vi "2D_Iteration_Data.vi"(9 "Iteration":i32, 10 "ID":dbl) -> (1 "y0":dbl, 2 "x0":dbl)   [LabVIEW 2011]
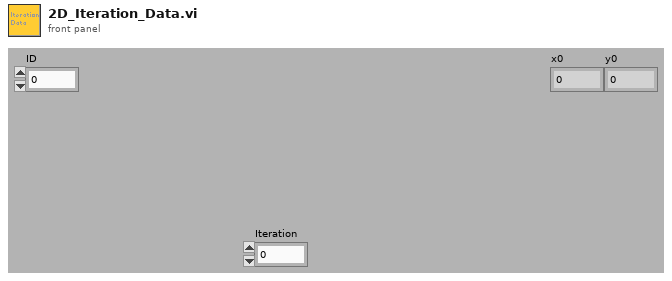
[diagram p1: front panel]
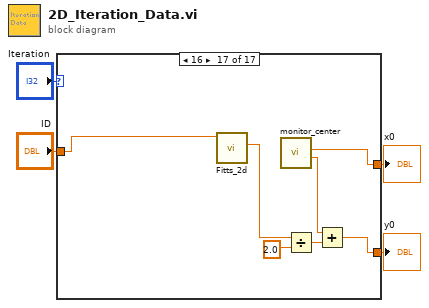
[diagram p0: block diagram]
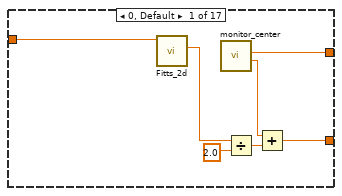
[diagram p2: hidden frame]
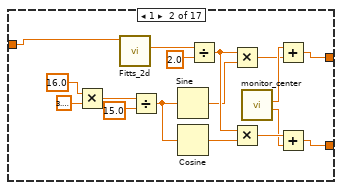
[diagram p3: hidden frame]
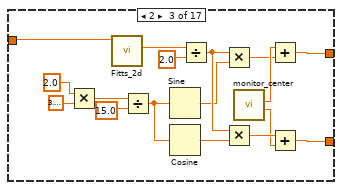
[diagram p4: hidden frame]
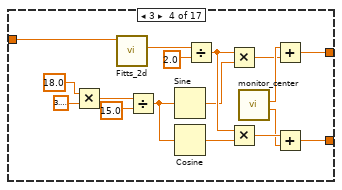
[diagram p5: hidden frame]
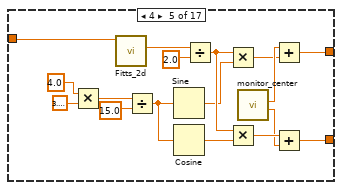
[diagram p6: hidden frame]
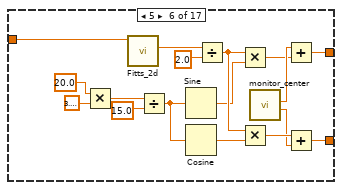
[diagram p7: hidden frame]
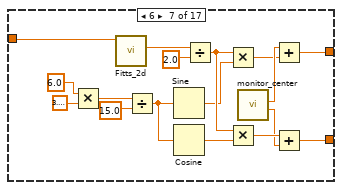
[diagram p8: hidden frame]
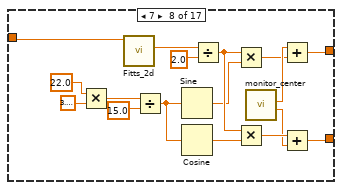
[diagram p9: hidden frame]
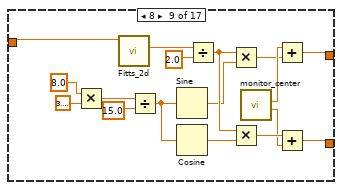
[diagram p10: hidden frame]
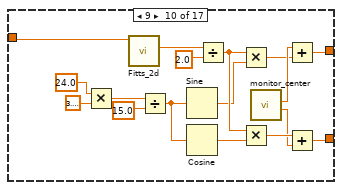
[diagram p11: hidden frame]
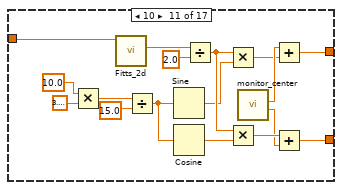
[diagram p12: hidden frame]
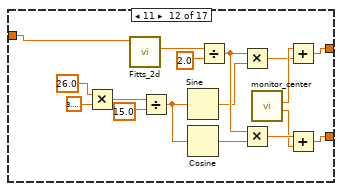
[diagram p13: hidden frame]
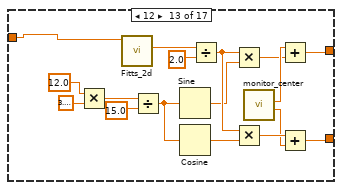
[diagram p14: hidden frame]
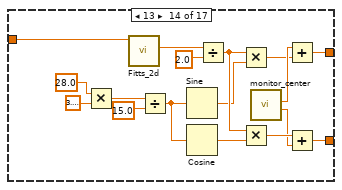
[diagram p15: hidden frame]
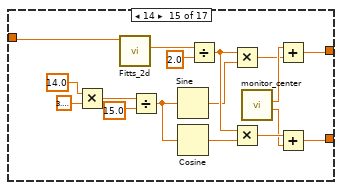
[diagram p16: hidden frame]
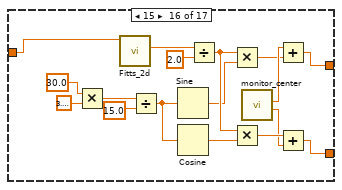
[diagram p17: hidden frame]
diagram:
  n1 = case shown="16" "Iteration" {
    tunnel: "ID" -> [w5 w14 w31 w48 w65 w82 w99 w116 w133 w150 w167 w184 w201 w218 w235 w252 w269]
    tunnel: [w7 w13 w30 w47 w64 w81 w98 w115 w132 w149 w166 w183 w200 w217 w234 w251 w268] -> w2
    tunnel: [w6 w12 w29 w46 w63 w80 w97 w114 w131 w148 w165 w182 w199 w216 w233 w250 w267] -> w1
    frame 0, Default {
      n2 = call "Fitts_2d.vi"("ID"=w5) -> ("D"=w10:dbl)  [unwired: 9 in, 1 out]
      n3 = call "monitor_center.vi"() -> ("yc"=w8:dbl, "xc"=w7:dbl)  [unwired: 10 in]
      n4 = Divide(x=w10, y=2.0) -> (x/y=w9:dbl)
      n5 = Add(x=w8, y=w9) -> (x+y=w6:dbl)
    }
    frame 1 {
      n6 = Multiply(x=16.0, y=3.141592653589793) -> (x*y=w15:dbl)
      n7 = call "Fitts_2d.vi"("ID"=w14) -> ("D"=w27:dbl)  [unwired: 9 in, 1 out]
      n8 = Divide(x=w15, y=15.0) -> (x/y=w24:dbl)
      n9 = Sine(x=w24) -> (sin(x)=w22:dbl)
      n10 = Cosine(x=w24) -> (cos(x)=w25:dbl)
      n11 = Divide(x=w27, y=2.0) -> (x/y=w23:dbl)
      n12 = Multiply(x=w23, y=w22) -> (x*y=w18:dbl)
      n13 = Multiply(x=w23, y=w25) -> (x*y=w21:dbl)
      n14 = call "monitor_center.vi"() -> ("yc"=w20:dbl, "xc"=w19:dbl)  [unwired: 10 in]
      n15 = Add(x=w19, y=w18) -> (x+y=w13:dbl)
      n16 = Add(x=w21, y=w20) -> (x+y=w12:dbl)
    }
    frame 2 {
      n17 = Multiply(x=2.0, y=3.141592653589793) -> (x*y=w32:dbl)
      n18 = call "Fitts_2d.vi"("ID"=w31) -> ("D"=w44:dbl)  [unwired: 9 in, 1 out]
      n19 = Divide(x=w32, y=15.0) -> (x/y=w41:dbl)
      n20 = Sine(x=w41) -> (sin(x)=w39:dbl)
      n21 = Cosine(x=w41) -> (cos(x)=w42:dbl)
      n22 = Divide(x=w44, y=2.0) -> (x/y=w40:dbl)
      n23 = Multiply(x=w40, y=w39) -> (x*y=w35:dbl)
      n24 = Multiply(x=w40, y=w42) -> (x*y=w38:dbl)
      n25 = call "monitor_center.vi"() -> ("yc"=w37:dbl, "xc"=w36:dbl)  [unwired: 10 in]
      n26 = Add(x=w36, y=w35) -> (x+y=w30:dbl)
      n27 = Add(x=w38, y=w37) -> (x+y=w29:dbl)
    }
    frame 3 {
      n28 = Multiply(x=18.0, y=3.141592653589793) -> (x*y=w49:dbl)
      n29 = call "Fitts_2d.vi"("ID"=w48) -> ("D"=w61:dbl)  [unwired: 9 in, 1 out]
      n30 = Divide(x=w49, y=15.0) -> (x/y=w58:dbl)
      n31 = Sine(x=w58) -> (sin(x)=w56:dbl)
      n32 = Cosine(x=w58) -> (cos(x)=w59:dbl)
      n33 = Divide(x=w61, y=2.0) -> (x/y=w57:dbl)
      n34 = Multiply(x=w57, y=w56) -> (x*y=w52:dbl)
      n35 = Multiply(x=w57, y=w59) -> (x*y=w55:dbl)
      n36 = call "monitor_center.vi"() -> ("yc"=w54:dbl, "xc"=w53:dbl)  [unwired: 10 in]
      n37 = Add(x=w53, y=w52) -> (x+y=w47:dbl)
      n38 = Add(x=w55, y=w54) -> (x+y=w46:dbl)
    }
    frame 4 {
      n39 = Multiply(x=4.0, y=3.141592653589793) -> (x*y=w66:dbl)
      n40 = call "Fitts_2d.vi"("ID"=w65) -> ("D"=w78:dbl)  [unwired: 9 in, 1 out]
      n41 = Divide(x=w66, y=15.0) -> (x/y=w75:dbl)
      n42 = Sine(x=w75) -> (sin(x)=w73:dbl)
      n43 = Cosine(x=w75) -> (cos(x)=w76:dbl)
      n44 = Divide(x=w78, y=2.0) -> (x/y=w74:dbl)
      n45 = Multiply(x=w74, y=w73) -> (x*y=w69:dbl)
      n46 = Multiply(x=w74, y=w76) -> (x*y=w72:dbl)
      n47 = call "monitor_center.vi"() -> ("yc"=w71:dbl, "xc"=w70:dbl)  [unwired: 10 in]
      n48 = Add(x=w70, y=w69) -> (x+y=w64:dbl)
      n49 = Add(x=w72, y=w71) -> (x+y=w63:dbl)
    }
    frame 5 {
      n50 = Multiply(x=20.0, y=3.141592653589793) -> (x*y=w83:dbl)
      n51 = call "Fitts_2d.vi"("ID"=w82) -> ("D"=w95:dbl)  [unwired: 9 in, 1 out]
      n52 = Divide(x=w83, y=15.0) -> (x/y=w92:dbl)
      n53 = Sine(x=w92) -> (sin(x)=w90:dbl)
      n54 = Cosine(x=w92) -> (cos(x)=w93:dbl)
      n55 = Divide(x=w95, y=2.0) -> (x/y=w91:dbl)
      n56 = Multiply(x=w91, y=w90) -> (x*y=w86:dbl)
      n57 = Multiply(x=w91, y=w93) -> (x*y=w89:dbl)
      n58 = call "monitor_center.vi"() -> ("yc"=w88:dbl, "xc"=w87:dbl)  [unwired: 10 in]
      n59 = Add(x=w87, y=w86) -> (x+y=w81:dbl)
      n60 = Add(x=w89, y=w88) -> (x+y=w80:dbl)
    }
    frame 6 {
      n61 = Multiply(x=6.0, y=3.141592653589793) -> (x*y=w100:dbl)
      n62 = call "Fitts_2d.vi"("ID"=w99) -> ("D"=w112:dbl)  [unwired: 9 in, 1 out]
      n63 = Divide(x=w100, y=15.0) -> (x/y=w109:dbl)
      n64 = Sine(x=w109) -> (sin(x)=w107:dbl)
      n65 = Cosine(x=w109) -> (cos(x)=w110:dbl)
      n66 = Divide(x=w112, y=2.0) -> (x/y=w108:dbl)
      n67 = Multiply(x=w108, y=w107) -> (x*y=w103:dbl)
      n68 = Multiply(x=w108, y=w110) -> (x*y=w106:dbl)
      n69 = call "monitor_center.vi"() -> ("yc"=w105:dbl, "xc"=w104:dbl)  [unwired: 10 in]
      n70 = Add(x=w104, y=w103) -> (x+y=w98:dbl)
      n71 = Add(x=w106, y=w105) -> (x+y=w97:dbl)
    }
    frame 7 {
      n72 = Multiply(x=22.0, y=3.141592653589793) -> (x*y=w117:dbl)
      n73 = call "Fitts_2d.vi"("ID"=w116) -> ("D"=w129:dbl)  [unwired: 9 in, 1 out]
      n74 = Divide(x=w117, y=15.0) -> (x/y=w126:dbl)
      n75 = Sine(x=w126) -> (sin(x)=w124:dbl)
      n76 = Cosine(x=w126) -> (cos(x)=w127:dbl)
      n77 = Divide(x=w129, y=2.0) -> (x/y=w125:dbl)
      n78 = Multiply(x=w125, y=w124) -> (x*y=w120:dbl)
      n79 = Multiply(x=w125, y=w127) -> (x*y=w123:dbl)
      n80 = call "monitor_center.vi"() -> ("yc"=w122:dbl, "xc"=w121:dbl)  [unwired: 10 in]
      n81 = Add(x=w121, y=w120) -> (x+y=w115:dbl)
      n82 = Add(x=w123, y=w122) -> (x+y=w114:dbl)
    }
    frame 8 {
      n83 = Multiply(x=8.0, y=3.141592653589793) -> (x*y=w134:dbl)
      n84 = call "Fitts_2d.vi"("ID"=w133) -> ("D"=w146:dbl)  [unwired: 9 in, 1 out]
      n85 = Divide(x=w134, y=15.0) -> (x/y=w143:dbl)
      n86 = Sine(x=w143) -> (sin(x)=w141:dbl)
      n87 = Cosine(x=w143) -> (cos(x)=w144:dbl)
      n88 = Divide(x=w146, y=2.0) -> (x/y=w142:dbl)
      n89 = Multiply(x=w142, y=w141) -> (x*y=w137:dbl)
      n90 = Multiply(x=w142, y=w144) -> (x*y=w140:dbl)
      n91 = call "monitor_center.vi"() -> ("yc"=w139:dbl, "xc"=w138:dbl)  [unwired: 10 in]
      n92 = Add(x=w138, y=w137) -> (x+y=w132:dbl)
      n93 = Add(x=w140, y=w139) -> (x+y=w131:dbl)
    }
    frame 9 {
      n94 = Multiply(x=24.0, y=3.141592653589793) -> (x*y=w151:dbl)
      n95 = call "Fitts_2d.vi"("ID"=w150) -> ("D"=w163:dbl)  [unwired: 9 in, 1 out]
      n96 = Divide(x=w151, y=15.0) -> (x/y=w160:dbl)
      n97 = Sine(x=w160) -> (sin(x)=w158:dbl)
      n98 = Cosine(x=w160) -> (cos(x)=w161:dbl)
      n99 = Divide(x=w163, y=2.0) -> (x/y=w159:dbl)
      n100 = Multiply(x=w159, y=w158) -> (x*y=w154:dbl)
      n101 = Multiply(x=w159, y=w161) -> (x*y=w157:dbl)
      n102 = call "monitor_center.vi"() -> ("yc"=w156:dbl, "xc"=w155:dbl)  [unwired: 10 in]
      n103 = Add(x=w155, y=w154) -> (x+y=w149:dbl)
      n104 = Add(x=w157, y=w156) -> (x+y=w148:dbl)
    }
    frame 10 {
      n105 = Multiply(x=10.0, y=3.141592653589793) -> (x*y=w168:dbl)
      n106 = call "Fitts_2d.vi"("ID"=w167) -> ("D"=w180:dbl)  [unwired: 9 in, 1 out]
      n107 = Divide(x=w168, y=15.0) -> (x/y=w177:dbl)
      n108 = Sine(x=w177) -> (sin(x)=w175:dbl)
      n109 = Cosine(x=w177) -> (cos(x)=w178:dbl)
      n110 = Divide(x=w180, y=2.0) -> (x/y=w176:dbl)
      n111 = Multiply(x=w176, y=w175) -> (x*y=w171:dbl)
      n112 = Multiply(x=w176, y=w178) -> (x*y=w174:dbl)
      n113 = call "monitor_center.vi"() -> ("yc"=w173:dbl, "xc"=w172:dbl)  [unwired: 10 in]
      n114 = Add(x=w172, y=w171) -> (x+y=w166:dbl)
      n115 = Add(x=w174, y=w173) -> (x+y=w165:dbl)
    }
    frame 11 {
      n116 = Multiply(x=26.0, y=3.141592653589793) -> (x*y=w185:dbl)
      n117 = call "Fitts_2d.vi"("ID"=w184) -> ("D"=w197:dbl)  [unwired: 9 in, 1 out]
      n118 = Divide(x=w185, y=15.0) -> (x/y=w194:dbl)
      n119 = Sine(x=w194) -> (sin(x)=w192:dbl)
      n120 = Cosine(x=w194) -> (cos(x)=w195:dbl)
      n121 = Divide(x=w197, y=2.0) -> (x/y=w193:dbl)
      n122 = Multiply(x=w193, y=w192) -> (x*y=w188:dbl)
      n123 = Multiply(x=w193, y=w195) -> (x*y=w191:dbl)
      n124 = call "monitor_center.vi"() -> ("yc"=w190:dbl, "xc"=w189:dbl)  [unwired: 10 in]
      n125 = Add(x=w189, y=w188) -> (x+y=w183:dbl)
      n126 = Add(x=w191, y=w190) -> (x+y=w182:dbl)
    }
    frame 12 {
      n127 = Multiply(x=12.0, y=3.141592653589793) -> (x*y=w202:dbl)
      n128 = call "Fitts_2d.vi"("ID"=w201) -> ("D"=w214:dbl)  [unwired: 9 in, 1 out]
      n129 = Divide(x=w202, y=15.0) -> (x/y=w211:dbl)
      n130 = Sine(x=w211) -> (sin(x)=w209:dbl)
      n131 = Cosine(x=w211) -> (cos(x)=w212:dbl)
      n132 = Divide(x=w214, y=2.0) -> (x/y=w210:dbl)
      n133 = Multiply(x=w210, y=w209) -> (x*y=w205:dbl)
      n134 = Multiply(x=w210, y=w212) -> (x*y=w208:dbl)
      n135 = call "monitor_center.vi"() -> ("yc"=w207:dbl, "xc"=w206:dbl)  [unwired: 10 in]
      n136 = Add(x=w206, y=w205) -> (x+y=w200:dbl)
      n137 = Add(x=w208, y=w207) -> (x+y=w199:dbl)
    }
    frame 13 {
      n138 = Multiply(x=28.0, y=3.141592653589793) -> (x*y=w219:dbl)
      n139 = call "Fitts_2d.vi"("ID"=w218) -> ("D"=w231:dbl)  [unwired: 9 in, 1 out]
      n140 = Divide(x=w219, y=15.0) -> (x/y=w228:dbl)
      n141 = Sine(x=w228) -> (sin(x)=w226:dbl)
      n142 = Cosine(x=w228) -> (cos(x)=w229:dbl)
      n143 = Divide(x=w231, y=2.0) -> (x/y=w227:dbl)
      n144 = Multiply(x=w227, y=w226) -> (x*y=w222:dbl)
      n145 = Multiply(x=w227, y=w229) -> (x*y=w225:dbl)
      n146 = call "monitor_center.vi"() -> ("yc"=w224:dbl, "xc"=w223:dbl)  [unwired: 10 in]
      n147 = Add(x=w223, y=w222) -> (x+y=w217:dbl)
      n148 = Add(x=w225, y=w224) -> (x+y=w216:dbl)
    }
    frame 14 {
      n149 = Multiply(x=14.0, y=3.141592653589793) -> (x*y=w236:dbl)
      n150 = call "Fitts_2d.vi"("ID"=w235) -> ("D"=w248:dbl)  [unwired: 9 in, 1 out]
      n151 = Divide(x=w236, y=15.0) -> (x/y=w245:dbl)
      n152 = Sine(x=w245) -> (sin(x)=w243:dbl)
      n153 = Cosine(x=w245) -> (cos(x)=w246:dbl)
      n154 = Divide(x=w248, y=2.0) -> (x/y=w244:dbl)
      n155 = Multiply(x=w244, y=w243) -> (x*y=w239:dbl)
      n156 = Multiply(x=w244, y=w246) -> (x*y=w242:dbl)
      n157 = call "monitor_center.vi"() -> ("yc"=w241:dbl, "xc"=w240:dbl)  [unwired: 10 in]
      n158 = Add(x=w240, y=w239) -> (x+y=w234:dbl)
      n159 = Add(x=w242, y=w241) -> (x+y=w233:dbl)
    }
    frame 15 {
      n160 = Multiply(x=30.0, y=3.141592653589793) -> (x*y=w253:dbl)
      n161 = call "Fitts_2d.vi"("ID"=w252) -> ("D"=w265:dbl)  [unwired: 9 in, 1 out]
      n162 = Divide(x=w253, y=15.0) -> (x/y=w262:dbl)
      n163 = Sine(x=w262) -> (sin(x)=w260:dbl)
      n164 = Cosine(x=w262) -> (cos(x)=w263:dbl)
      n165 = Divide(x=w265, y=2.0) -> (x/y=w261:dbl)
      n166 = Multiply(x=w261, y=w260) -> (x*y=w256:dbl)
      n167 = Multiply(x=w261, y=w263) -> (x*y=w259:dbl)
      n168 = call "monitor_center.vi"() -> ("yc"=w258:dbl, "xc"=w257:dbl)  [unwired: 10 in]
      n169 = Add(x=w257, y=w256) -> (x+y=w251:dbl)
      n170 = Add(x=w259, y=w258) -> (x+y=w250:dbl)
    }
    frame 16 {
      n171 = call "Fitts_2d.vi"("ID"=w269) -> ("D"=w272:dbl)  [unwired: 9 in, 1 out]
      n172 = call "monitor_center.vi"() -> ("yc"=w270:dbl, "xc"=w268:dbl)  [unwired: 10 in]
      n173 = Divide(x=w272, y=2.0) -> (x/y=w271:dbl)
      n174 = Add(x=w270, y=w271) -> (x+y=w267:dbl)
    }
  }
  "x0" <- w2
  "y0" <- w1
